vi "AVS_Measure.vi"(0 "a_hDevice":i32, 7 "a_hWnd":i32, 11 "a_Nmsr":i16) -> (4 "Output Value":i32)   [LabVIEW 2020]
uses:
  AvaSpecX64-DLL_9.4/avaspecx64.dll
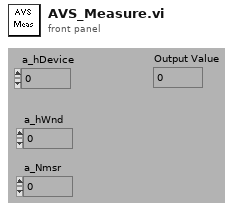
[diagram p1: front panel]
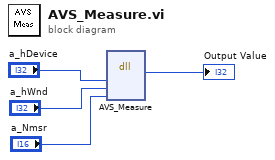
[diagram p0: block diagram]
diagram:
  n1 = dll-call lib="C:/AvaSpecX64-DLL_9.4/avaspecx64.dll" fn="AVS_Measure"("a_hDevice"="a_hDevice", "a_hWnd"="a_hWnd", "a_Nmsr"="a_Nmsr") -> ("return type"=→"Output Value":i32)  [unwired: 6 in, 2 out]
